vi "Select String Based on OS.vi"(10 "Strings":T1) -> (2 "Selection":string)   [LabVIEW 2020, in "Approval Tests.lvlib"]
uses:
  Approval Tests.lvlib
  OS Strings.ctl
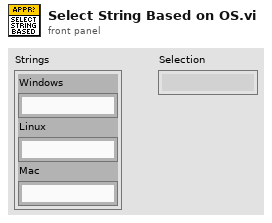
[diagram p1: front panel]
types:
  T1 = typedef "Approval Tests.lvlib/OS Strings.ctl" = cluster{"Windows":string, "Linux":string, "Mac":string}
  T2 = enum32{"invalid OS target", "Mac OS", "Windows 3.1", "Windows 95/NT", "Solaris 1", "Solaris 2", "HP-UX", "PowerMAX", "Linux", "Irix", "Rhapsody", "BeOS", "AIX", "OSF1", "VxWorks", "PharLap", "Carbon", "RTX", "Windows x64", "Linux x64", "Mac OS X x64", "Linux ARM64", "Windows ARM64", "Mac OS X ARM64"}
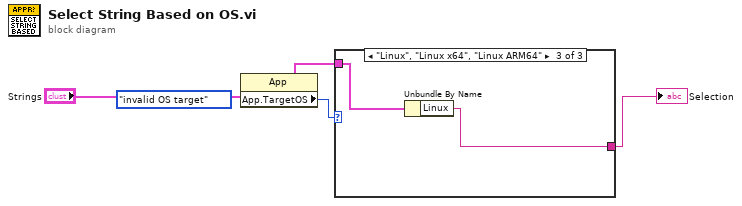
[diagram p0: block diagram]
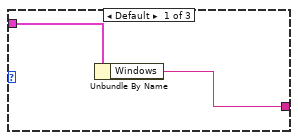
[diagram p2: hidden frame]
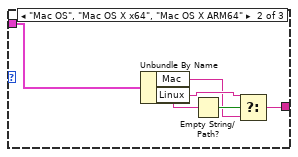
[diagram p3: hidden frame]
diagram:
  (unwired) T2."invalid OS target" ("Application:Target:Operating System")
  n1 = property class="App"() -> ("App.TargetOS"=w3:T2)  [unwired: 2 in, 2 out]
  n2 = case shown="\"Linux\", \"Linux x64\", \"Linux ARM64\"" w3 {
    tunnel: "Strings" -> [w5 w10 w12]
    tunnel: [w4 w6 w11] -> w1
    frame Default {
      n3 = Unbundle By Name(w5) -> ("Windows"=w4:string)
    }
    frame "Mac OS", "Mac OS X x64", "Mac OS X ARM64" {
      n4 = Unbundle By Name(w10) -> ("Mac"=w7:string, "Linux"=w8:string)
      n5 = Empty String/Path?(string/path=w7) -> (empty?=w9:bool)
      n6 = Select(t=w8, s=w9, f=w7) -> (s? t:f=w6:string)
    }
    frame "Linux", "Linux x64", "Linux ARM64" {
      n7 = Unbundle By Name(w12) -> ("Linux"=w11:string)
    }
  }
  "Selection" <- w1
